vi "Create Points for a Unit Circle.vi"() -> (0 "Cluster":cluster{dbl[], dbl[]})   [LabVIEW 2010, in "Core SubVIs.lvlib"]
uses:
  Core SubVIs.lvlib
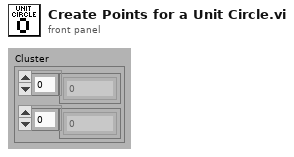
[diagram p1: front panel]
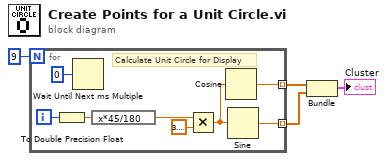
[diagram p0: block diagram]
diagram:
  n1 = for {
    N: 9 -> [_]
    tunnel: [w7] -> w2 mode=indexing
    tunnel: [w6] -> w3 mode=indexing
    i -> [w12]
    # "Calculate Unit Circle for Display"
    n2 = To Double Precision Float(number=w12) -> (double precision float=w11:dbl)
    n3 = Wait Until Next ms Multiple(millisecond multiple=u32 0) -> ()  [unwired: 1 out]
    n4 = expression code="x*45/180"(w11) -> (w10:dbl)
    n5 = Multiply(x=w10, y=3.141592653589793) -> (x*y=w8:dbl)
    n6 = Cosine(x=w8) -> (cos(x)=w7:dbl)
    n7 = Sine(x=w8) -> (sin(x)=w6:dbl)
  }
  n8 = Bundle(w2, w3) -> (→"Cluster":cluster{dbl[], dbl[]})  [unwired: 1 in]
